vi "SetupColumns.vi"(0 "reference in":refnum<class "DataGridView.lvclass">, 5 "ColumnSettings":T1[](array[typedef]) {"Width" min=2 step=1; "MinWidth" min=2 step=1; "AutoSizeMode" items=["None"=1, "ColumnHeader"=2, "AllCellsExceptHeader"=4, "AllCells"=6, "DisplayedCellsExceptHeader"=8, "DisplayedCells"=10, "Fill"=16]; "FillWeight" min=2 step=1}, 11 "error in (no error)":errorcluster) -> (4 "reference out":refnum<class "DataGridView.lvclass">, 15 "error out":errorcluster)   [LabVIEW 2018, in "DataGridView.lvclass"]
doc: "Used to setup the columns of the DataGridView, here you can set if a column should be a text, combobox, timestamp or image column"
uses:
  DataGridView.lvclass
  typedefs/ColumSetting.ctl
  typedefs/ColumnType.ctl
  System.Windows.Forms
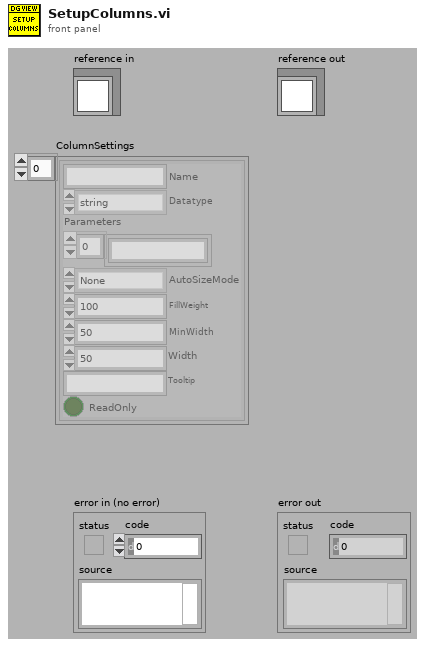
[diagram p1: front panel]
types:
  T1 = typedef "DataGridView.lvclass/ColumSetting.ctl" = cluster{"Name":string, "Datatype":T2, "Parameters":string[], "AutoSizeMode":i32, "FillWeight":sgl, "MinWidth":u32, "Width":u32, "Tooltip":string, "ReadOnly":bool}
  T2 = typedef "DataGridView.lvclass/ColumnType.ctl" = enum16{"string", "image", "check", "numeric", "timestamp", "button", "combo", "link"}
  T3 = typedef "DataGridView.lvclass/ObjectAttributes.ctl" = cluster{"DataGridView":refnum<k24>, "SelectionChangedEvent":refnum<user-event>, "SelectionChanged callback ref":refnum<k27>, "LastSelectedRowIndex":i32}
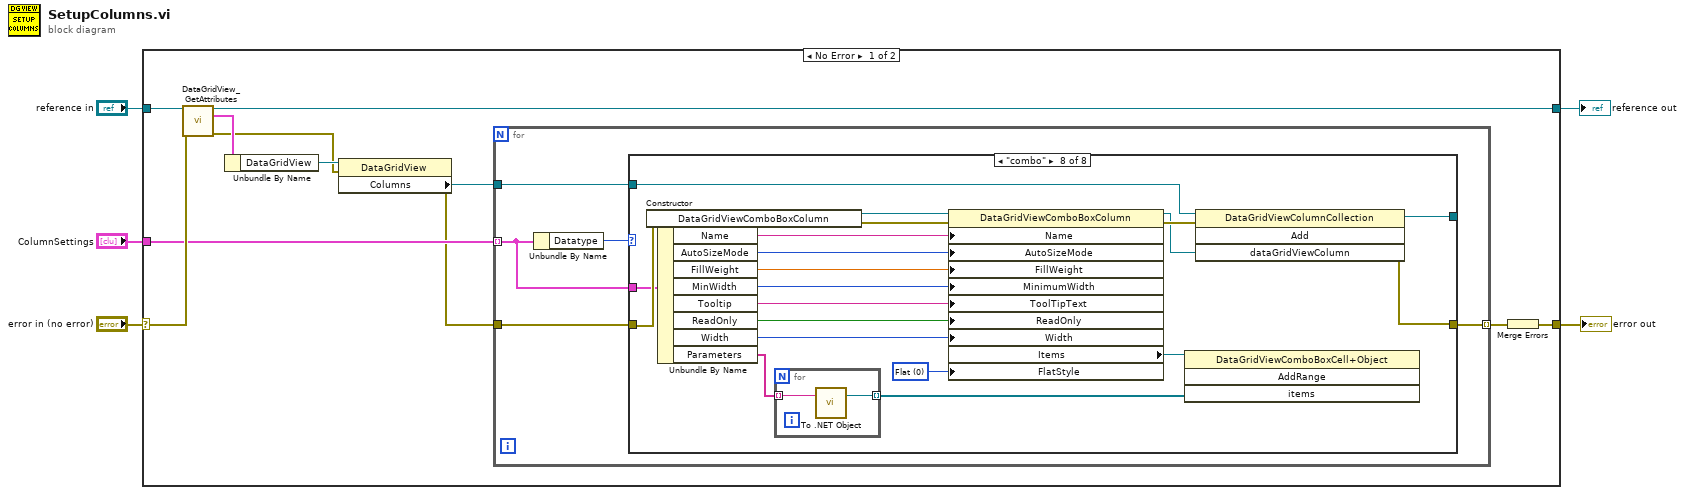
[diagram p0: block diagram]
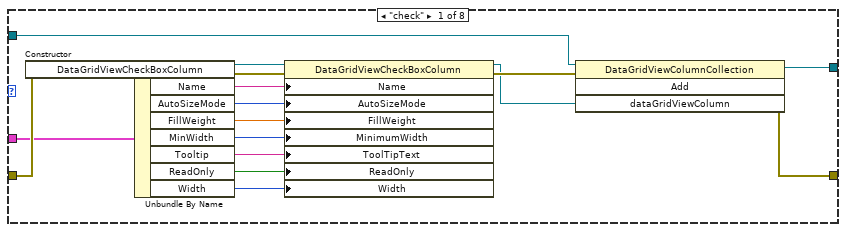
[diagram p2: hidden frame]
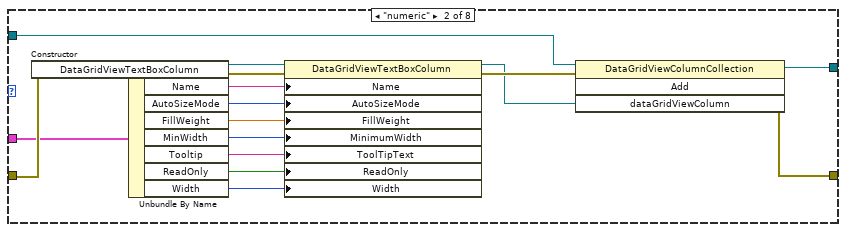
[diagram p3: hidden frame]
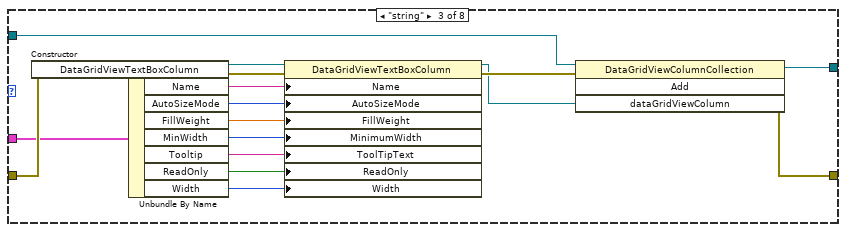
[diagram p4: hidden frame]
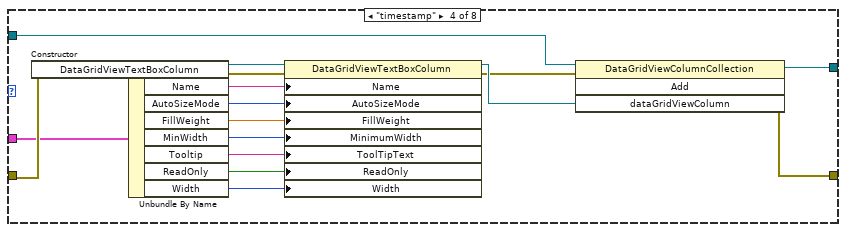
[diagram p5: hidden frame]
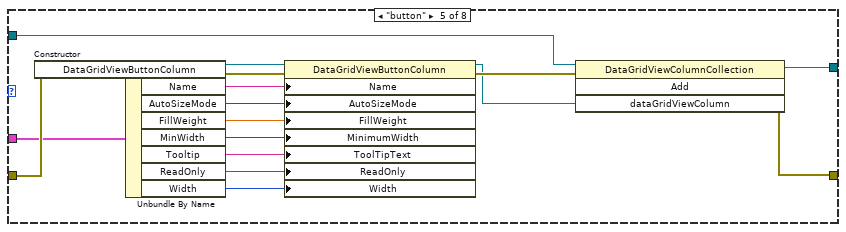
[diagram p6: hidden frame]
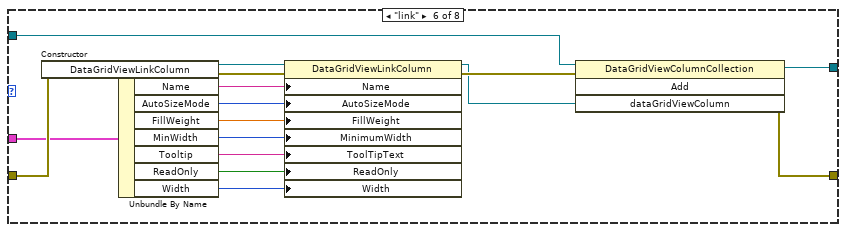
[diagram p7: hidden frame]
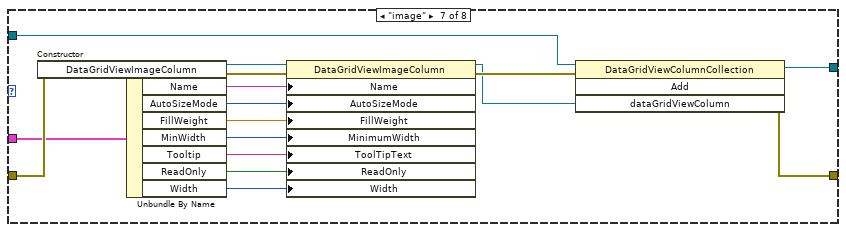
[diagram p8: hidden frame]
diagram:
  n1 = case shown="No Error" "error in (no error)" {
    selector: "error in (no error)" -> [w16 w157]
    tunnel: [w7 w157] -> w4
    tunnel: [w13 w156] -> w2
    tunnel: "reference in" -> [w14 w156]
    tunnel: "ColumnSettings" -> [w11 _]
    frame No Error {
      n2 = call "DataGridView_GetAttributes.vi"("reference in"=w14, "error in (no error)"=w16) -> ("reference out"=w13:refnum<class "DataGridView.lvclass">, "Data"=w15:T3, "error out"=w10:errorcluster)  [unwired: 10 in, 1 out]
      n3 = Unbundle By Name(w15) -> ("DataGridView"=w12:refnum<k24>)
      n4 = property class="DataGridView"(reference=w12, error in=w10) -> (error out=w9:errorcluster, "Columns"=w8:refnum<k24>)  [unwired: 1 out]
      n5 = for {
        tunnel: w11 -> [w17] mode=indexing
        tunnel: w9 -> [w18]
        tunnel: w8 -> [w21]
        tunnel: [w19] -> w6 mode=indexing
        n6 = Unbundle By Name(w17) -> ("Datatype"=w20:T2)
        n7 = case shown="\"combo\"" w20 {
          tunnel: [w37 w52 w69 w85 w101 w117 w133 w153] -> _
          tunnel: w21 -> [w36 w51 w68 w84 w100 w116 w132 w152]
          tunnel: [w34 w49 w66 w82 w98 w114 w130 w151] -> w19
          tunnel: w18 -> [w35 w50 w67 w83 w99 w115 w131 w150]
          tunnel: w17 -> [w27 w45 w59 w75 w87 w103 w123 w140]
          frame "check" {
            n8 = constructor class="DataGridViewCheckBoxColumn"(error in=w35) -> (reference out=w25:refnum<k24>, error out=w26:errorcluster)  [unwired: 2 in, 1 out]
            n9 = Unbundle By Name(w27) -> ("Name"=w33:string, "AutoSizeMode"=w32:i32, "FillWeight"=w31:sgl, "MinWidth"=w30:u32, "Tooltip"=w29:string, "ReadOnly"=w28:bool, "Width"=w22:u32)
            n10 = property class="DataGridViewCheckBoxColumn"(reference=w25, error in=w26, "Name"=w33, "AutoSizeMode"=w32, "FillWeight"=w31, "MinimumWidth"=w30, "ToolTipText"=w29, "ReadOnly"=w28, "Width"=w22) -> (reference out=w23:refnum<k24>, error out=w24:errorcluster)
            n11 = invoke class="DataGridViewColumnCollection" method="Add"(reference=w36, error in=w24, "dataGridViewColumn"=w23) -> (reference out=w37:refnum<k24>, error out=w34:errorcluster)  [unwired: 1 in, 2 out]
          }
          frame "numeric" {
            n12 = constructor class="DataGridViewTextBoxColumn"(error in=w50) -> (reference out=w47:refnum<k24>, error out=w53:errorcluster)  [unwired: 2 in, 1 out]
            n13 = Unbundle By Name(w45) -> ("Name"=w44:string, "AutoSizeMode"=w43:i32, "FillWeight"=w42:sgl, "MinWidth"=w41:u32, "Tooltip"=w40:string, "ReadOnly"=w39:bool, "Width"=w38:u32)
            n14 = property class="DataGridViewTextBoxColumn"(reference=w47, error in=w53, "Name"=w44, "AutoSizeMode"=w43, "FillWeight"=w42, "MinimumWidth"=w41, "ToolTipText"=w40, "ReadOnly"=w39, "Width"=w38) -> (reference out=w46:refnum<k24>, error out=w48:errorcluster)
            n15 = invoke class="DataGridViewColumnCollection" method="Add"(reference=w51, error in=w48, "dataGridViewColumn"=w46) -> (reference out=w52:refnum<k24>, error out=w49:errorcluster)  [unwired: 1 in, 2 out]
          }
          frame "string" {
            n16 = constructor class="DataGridViewTextBoxColumn"(error in=w67) -> (reference out=w58:refnum<k24>, error out=w57:errorcluster)  [unwired: 2 in, 1 out]
            n17 = Unbundle By Name(w59) -> ("Name"=w65:string, "AutoSizeMode"=w64:i32, "FillWeight"=w63:sgl, "MinWidth"=w62:u32, "Tooltip"=w61:string, "ReadOnly"=w60:bool, "Width"=w54:u32)
            n18 = property class="DataGridViewTextBoxColumn"(reference=w58, error in=w57, "Name"=w65, "AutoSizeMode"=w64, "FillWeight"=w63, "MinimumWidth"=w62, "ToolTipText"=w61, "ReadOnly"=w60, "Width"=w54) -> (reference out=w55:refnum<k24>, error out=w56:errorcluster)
            n19 = invoke class="DataGridViewColumnCollection" method="Add"(reference=w68, error in=w56, "dataGridViewColumn"=w55) -> (reference out=w69:refnum<k24>, error out=w66:errorcluster)  [unwired: 1 in, 2 out]
          }
          frame "timestamp" {
            n20 = constructor class="DataGridViewTextBoxColumn"(error in=w83) -> (reference out=w74:refnum<k24>, error out=w73:errorcluster)  [unwired: 2 in, 1 out]
            n21 = Unbundle By Name(w75) -> ("Name"=w81:string, "AutoSizeMode"=w80:i32, "FillWeight"=w79:sgl, "MinWidth"=w78:u32, "Tooltip"=w77:string, "ReadOnly"=w76:bool, "Width"=w70:u32)
            n22 = property class="DataGridViewTextBoxColumn"(reference=w74, error in=w73, "Name"=w81, "AutoSizeMode"=w80, "FillWeight"=w79, "MinimumWidth"=w78, "ToolTipText"=w77, "ReadOnly"=w76, "Width"=w70) -> (reference out=w72:refnum<k24>, error out=w71:errorcluster)
            n23 = invoke class="DataGridViewColumnCollection" method="Add"(reference=w84, error in=w71, "dataGridViewColumn"=w72) -> (reference out=w85:refnum<k24>, error out=w82:errorcluster)  [unwired: 1 in, 2 out]
          }
          frame "button" {
            n24 = constructor class="DataGridViewButtonColumn"(error in=w99) -> (reference out=w90:refnum<k24>, error out=w91:errorcluster)  [unwired: 2 in, 1 out]
            n25 = Unbundle By Name(w87) -> ("Name"=w97:string, "AutoSizeMode"=w96:i32, "FillWeight"=w95:sgl, "MinWidth"=w94:u32, "Tooltip"=w93:string, "ReadOnly"=w92:bool, "Width"=w86:u32)
            n26 = property class="DataGridViewButtonColumn"(reference=w90, error in=w91, "Name"=w97, "AutoSizeMode"=w96, "FillWeight"=w95, "MinimumWidth"=w94, "ToolTipText"=w93, "ReadOnly"=w92, "Width"=w86) -> (reference out=w88:refnum<k24>, error out=w89:errorcluster)
            n27 = invoke class="DataGridViewColumnCollection" method="Add"(reference=w100, error in=w89, "dataGridViewColumn"=w88) -> (reference out=w101:refnum<k24>, error out=w98:errorcluster)  [unwired: 1 in, 2 out]
          }
          frame "link" {
            n28 = constructor class="DataGridViewLinkColumn"(error in=w115) -> (reference out=w106:refnum<k24>, error out=w107:errorcluster)  [unwired: 2 in, 1 out]
            n29 = Unbundle By Name(w103) -> ("Name"=w113:string, "AutoSizeMode"=w112:i32, "FillWeight"=w111:sgl, "MinWidth"=w110:u32, "Tooltip"=w109:string, "ReadOnly"=w108:bool, "Width"=w102:u32)
            n30 = property class="DataGridViewLinkColumn"(reference=w106, error in=w107, "Name"=w113, "AutoSizeMode"=w112, "FillWeight"=w111, "MinimumWidth"=w110, "ToolTipText"=w109, "ReadOnly"=w108, "Width"=w102) -> (reference out=w104:refnum<k24>, error out=w105:errorcluster)
            n31 = invoke class="DataGridViewColumnCollection" method="Add"(reference=w116, error in=w105, "dataGridViewColumn"=w104) -> (reference out=w117:refnum<k24>, error out=w114:errorcluster)  [unwired: 1 in, 2 out]
          }
          frame "image" {
            n32 = constructor class="DataGridViewImageColumn"(error in=w131) -> (reference out=w121:refnum<k24>, error out=w122:errorcluster)  [unwired: 2 in, 1 out]
            n33 = Unbundle By Name(w123) -> ("Name"=w129:string, "AutoSizeMode"=w128:i32, "FillWeight"=w127:sgl, "MinWidth"=w126:u32, "Tooltip"=w125:string, "ReadOnly"=w124:bool, "Width"=w118:u32)
            n34 = property class="DataGridViewImageColumn"(reference=w121, error in=w122, "Name"=w129, "AutoSizeMode"=w128, "FillWeight"=w127, "MinimumWidth"=w126, "ToolTipText"=w125, "ReadOnly"=w124, "Width"=w118) -> (reference out=w119:refnum<k24>, error out=w120:errorcluster)
            n35 = invoke class="DataGridViewColumnCollection" method="Add"(reference=w132, error in=w120, "dataGridViewColumn"=w119) -> (reference out=w133:refnum<k24>, error out=w130:errorcluster)  [unwired: 1 in, 2 out]
          }
          frame "combo" {
            w134 = 0 items=["Flat", "Popup", "Standard", "System"] ("FlatStyle")
            n36 = constructor class="DataGridViewComboBoxColumn"(error in=w150) -> (reference out=w142:refnum<k24>, error out=w143:errorcluster)  [unwired: 2 in, 1 out]
            n37 = Unbundle By Name(w140) -> ("Name"=w149:string, "AutoSizeMode"=w148:i32, "FillWeight"=w147:sgl, "MinWidth"=w146:u32, "Tooltip"=w145:string, "ReadOnly"=w144:bool, "Width"=w135:u32, "Parameters"=w137:string[])
            n38 = for {
              tunnel: w137 -> [w155] mode=indexing
              tunnel: [w154] -> w138 mode=indexing
              n39 = call <vilib>:"To .NET Object.vi"("anything"=w155) -> (".NET object"=w154:refnum<k24>)  [unwired: 1 in, 1 out]
            }
            n40 = property class="DataGridViewComboBoxColumn"(reference=w142, error in=w143, "Name"=w149, "AutoSizeMode"=w148, "FillWeight"=w147, "MinimumWidth"=w146, "ToolTipText"=w145, "ReadOnly"=w144, "Width"=w135, "FlatStyle"=w134) -> (reference out=w139:refnum<k24>, error out=w141:errorcluster, "Items"=w136:refnum<k24>)
            n41 = invoke class="DataGridViewComboBoxCell+Object" method="AddRange"(reference=w136, "items"=w138) -> ()  [unwired: 2 in, 4 out]
            n42 = invoke class="DataGridViewColumnCollection" method="Add"(reference=w152, error in=w141, "dataGridViewColumn"=w139) -> (reference out=w153:refnum<k24>, error out=w151:errorcluster)  [unwired: 1 in, 2 out]
          }
        }
      }
      n43 = Merge Errors(w6) -> (w7:errorcluster)
    }
    frame Error {
    }
  }
  "error out" <- w4
  "reference out" <- w2
